vi "Main.vi"() -> ()   [LabVIEW 2024, in "Word Search Scorer.lvlib"]
uses:
  Word Search Scorer.lvlib
  Result.ctl
panel:
  in  "Result":T1
  out "Response":string
  out "Upload Debug":string
  in  "Skip":bool
  in  "Upload":bool
  out "Completed":bool
  out "Run Time":dbl format="%_6f"
  in  "Cancel":bool
  in  "Run":bool
  out "Download Debug":string
  out "Get Next Debug":string
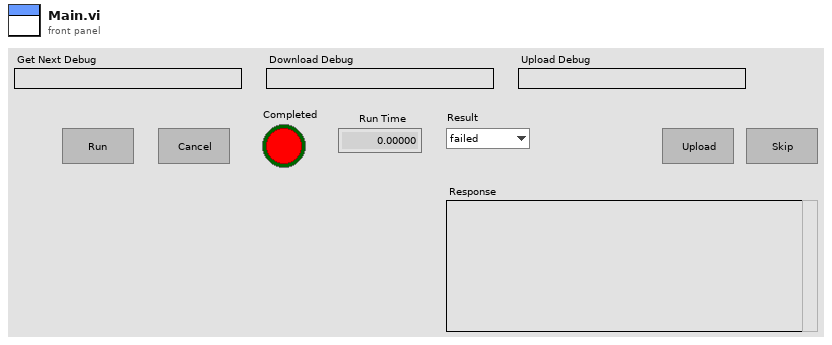
[diagram p1: front panel]
types:
  T1 = typedef "Word Search Scorer.lvlib/Result.ctl" = enum16{"failed", "complete", "error"}
  T2 = enum8{"Enabled", "Disabled", "Disabled and Grayed Out"}
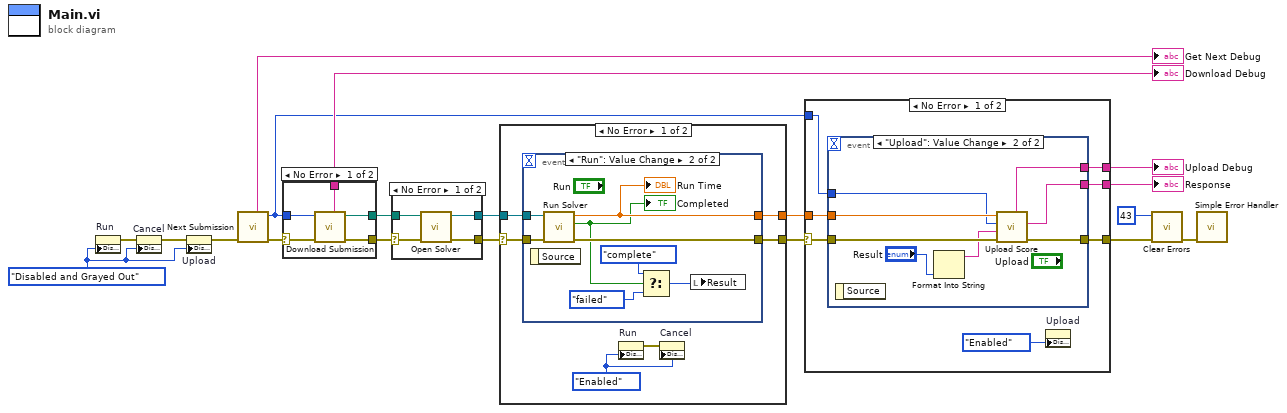
[diagram p0: block diagram]
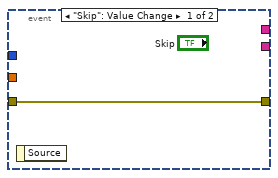
[diagram p2: hidden frame]
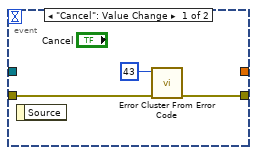
[diagram p6: hidden frame]
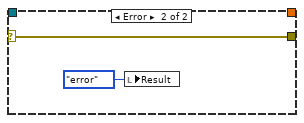
[diagram p7: hidden frame]
diagram:
  w8 = T2."Disabled and Grayed Out" ("Disabled")
  n1 = property on="Run" class="Bool"("DisabledEnum"=w8) -> (error out=w11:errorcluster)  [unwired: 2 in, 1 out]
  n2 = property on="Cancel" class="Bool"(error in=w11, "DisabledEnum"=w8) -> (error out=w10:errorcluster)  [unwired: 1 in, 1 out]
  n3 = property on="Upload" class="Bool"(error in=w10, "DisabledEnum"=w8) -> (error out=w9:errorcluster)  [unwired: 1 in, 1 out]
  n4 = call "Next Submission.vi"("error in (no error)"=w9) -> ("error out"=w18:errorcluster, "submission"=w3:i32, "Profile URL"=→"Get Next Debug":string)  [unwired: 8 in]
  n5 = case shown="No Error" w18 {
    selector: w18 -> [w23 w25]
    tunnel: w3 -> [w24 _]
    tunnel: [w22 _] -> w17
    tunnel: [w21 _] -> w15
    tunnel: [w20 w25] -> w16
    frame No Error {
      n6 = call "Download Submission.vi"("error in (no error)"=w23, "submission"=w24) -> ("error out"=w20:errorcluster, "Zip Path"=w21:path, "Profile URL"=w22:string)  [unwired: 7 in]
    }
    frame Error {
    }
  }
  "Download Debug" <- w17
  n7 = case shown="No Error" w16 {
    selector: w16 -> [w28 w30]
    tunnel: w15 -> [w29 _]
    tunnel: [w27 _] -> w14
    tunnel: [w26 w30] -> w13
    frame No Error {
      n8 = call "Open Solver.vi"("error in (no error)"=w28, "Solver Path"=w29) -> ("error IO"=w26:errorcluster, "Solver VI"=w27:refnum<vi>)  [unwired: 8 in]
    }
    frame Error {
    }
  }
  n9 = case shown="No Error" w13 {
    selector: w13 -> [w35 w49]
    tunnel: w14 -> [w36 _]
    tunnel: [w34 w49] -> w12
    tunnel: [w31 _] -> w4
    frame No Error {
      w33 = T2."Enabled" ("Disabled")
      n10 = event shown="[1] \"Run\": Value Change" {
        selector: _ -> [_ _]
        dyn-events: _ -> [_ _]
        timeout: _ -> [_ _]
        tunnel: w36 -> [_ w47]
        tunnel: w35 -> [w39 w46]
        tunnel: [w37 w45] -> w34
        tunnel: [_ w44] -> w31
        event "Cancel": Value Change {
          n11 = event-data() -> ()  [unwired: 1 in, 1 out]
          n12 = call <vilib>:"Error Cluster From Error Code.vi"("error in (no error)"=w39, "error code (0)"=43) -> ("error out"=w37:errorcluster)  [unwired: 7 in]
        }
        event "Run": Value Change {
          n13 = event-data() -> ()  [unwired: 1 in, 1 out]
          n14 = call "Run Solver.vi"("error in (no error)"=w46, "Solver VI"=w47) -> ("error out"=w45:errorcluster, "Completed"=w43:bool, "Run Time"=w44:dbl)  [unwired: 7 in]
          "Run Time" <- w44
          "Completed" <- w43
          n15 = Select(t=Result."complete" ("Result"), s=w43, f=Result."failed" ("Result")) -> (s? t:f=w41:T1)
          n16 = local write "Result"(w41) -> ()
        }
      }
      n17 = property on="Run" class="Bool"("DisabledEnum"=w33) -> (error out=w32:errorcluster)  [unwired: 2 in, 1 out]
      n18 = property on="Cancel" class="Bool"(error in=w32, "DisabledEnum"=w33) -> ()  [unwired: 1 in, 2 out]
    }
    frame Error {
      n19 = local write "Result"(Result."error" ("Result")) -> ()
    }
  }
  n20 = case shown="No Error" w12 {
    selector: w12 -> [w55 w66]
    tunnel: [w54 w66] -> w7
    tunnel: w4 -> [w53 _]
    tunnel: w3 -> [w52 _]
    tunnel: [w51 _] -> w2
    tunnel: [w50 _] -> w1
    frame No Error {
      n21 = event shown="[1] \"Upload\": Value Change" {
        selector: _ -> [_ _]
        dyn-events: _ -> [_ _]
        timeout: _ -> [_ _]
        tunnel: w55 -> [w57 w65]
        tunnel: [w57 w62] -> w54
        tunnel: w53 -> [_ w64]
        tunnel: w52 -> [_ w63]
        tunnel: [_ w61] -> w51
        tunnel: [_ w60] -> w50
        event "Skip": Value Change {
          n22 = event-data() -> ()  [unwired: 1 in, 1 out]
        }
        event "Upload": Value Change {
          n23 = event-data() -> ()  [unwired: 1 in, 1 out]
          n24 = Format Into String("Result") -> (resulting string=w58:string)  [unwired: 3 in, 1 out]
          n25 = call "Upload Score.vi"("error in (no error)"=w65, "status"=w58, "submission"=w63, "Run Time"=w64) -> ("error out"=w62:errorcluster, "Response"=w60:string, "Profile URL"=w61:string)  [unwired: 5 in]
        }
      }
      n26 = property on="Upload" class="Bool"("DisabledEnum"=T2."Enabled" ("Disabled")) -> ()  [unwired: 2 in, 2 out]
    }
    frame Error {
    }
  }
  "Upload Debug" <- w2
  "Response" <- w1
  n27 = call <vilib>:"Clear Errors.vi"("error in (no error)"=w7, "specific error code to clear (0: all)"=43) -> ("error out"=w6:errorcluster)  [unwired: 4 in, 1 out]
  n28 = call <vilib>:"Simple Error Handler.vi"("error in (no error)"=w6) -> ()  [unwired: 4 in, 5 out]
